vi "FTW-Message-ReadMetadata.vi"(0 "Message":refnum<class "FTW-Message.lvclass">, 11 "error in":errorcluster) -> (4 "Message out":refnum<class "FTW-Message.lvclass">, 6 "Tick Count":u32, 8 "Timestamp":timestamp format="%^<%Y-%m-%dT%H:%M:%S%3uZ>T", 15 "error out":errorcluster)   [LabVIEW 2014, in "FTW-Message.lvclass"]
uses:
  FTW-Message.lvclass
panel:
  # "Inputs"
  # "Outputs"
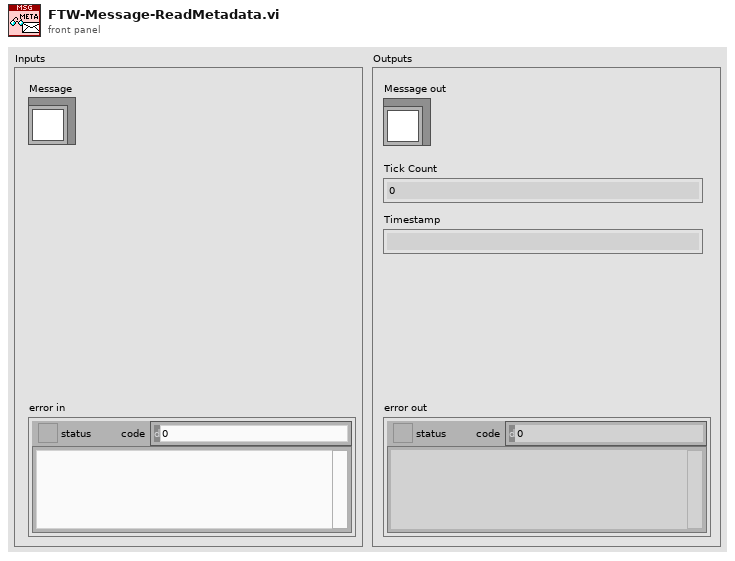
[diagram p1: front panel]
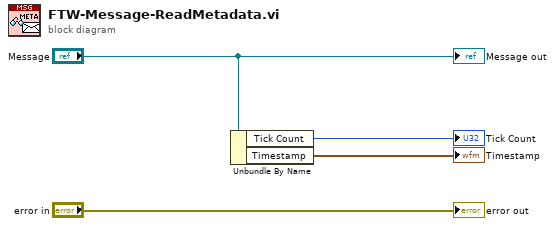
[diagram p0: block diagram]
diagram:
  n1 = Unbundle By Name("Message") -> ("Tick Count"=→"Tick Count":u32, "Timestamp"=→"Timestamp":timestamp)
  "error out" <- "error in"
  "Message out" <- "Message"
